vi "AB_Set_Library_Name_For_Destination.vi"(7 "allow empty string? (false)":bool, 8 "error in (no error)":errorcluster, 9 "library name":string, 10 "destination index":i32, 11 "destinations in":refnum<class "AB_Destination.lvclass">[](array[class])) -> (0 "error out":errorcluster, 2 "library name out":string, 3 "destinations out":refnum<class "AB_Destination.lvclass">[](array[class]))   [LabVIEW 2020]
uses:
  <vilib>/AppBuilder/AB_Classes/Destination/AB_Destination.lvclass
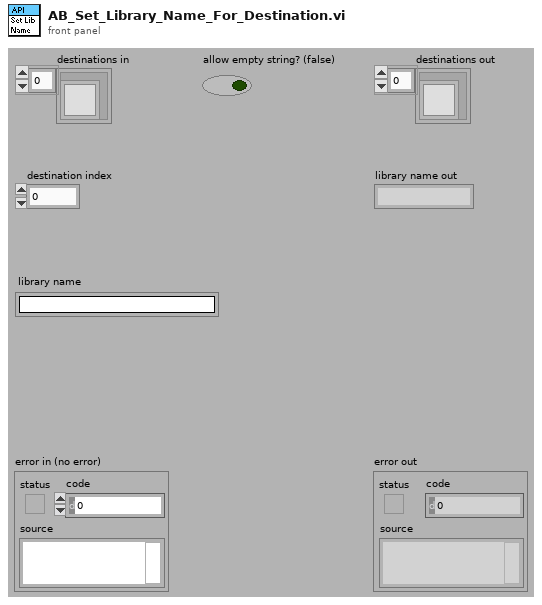
[diagram p1: front panel]
types:
  T1 = typedef "AB_Destination.ctl" = cluster{"destName":string, "path":path, "libraryName":string, "preserveHierarchy":bool, "eng_inBuild":bool, "eng_libraryReference":refnum<vi>, "eng_restictAddToNewLibrary":bool}
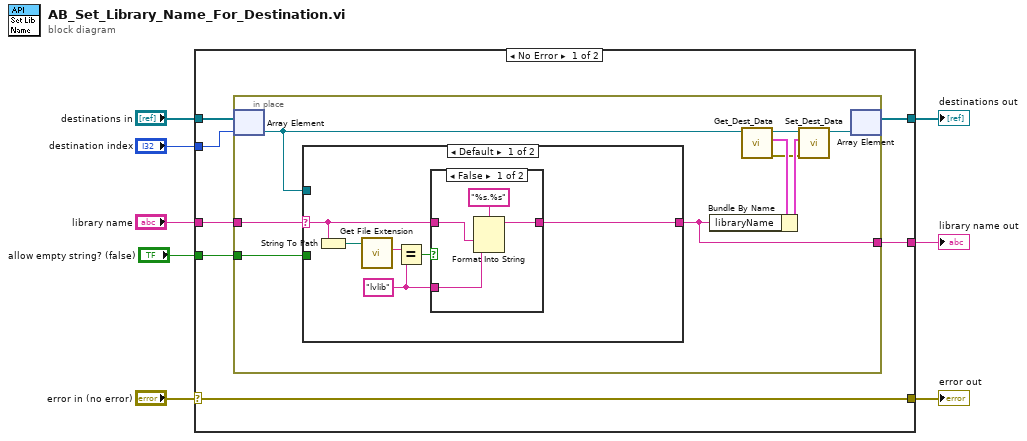
[diagram p0: block diagram]
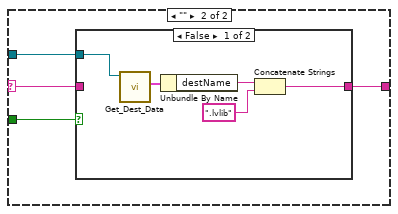
[diagram p3: hidden frame]
diagram:
  n1 = case shown="No Error" "error in (no error)" {
    selector: "error in (no error)" -> [w12 w47]
    tunnel: [w12 w47] -> w7
    tunnel: "destinations in" -> [w15 w46]
    tunnel: [w14 w46] -> w5
    tunnel: "destination index" -> [w13 _]
    tunnel: "library name" -> [w11 _]
    tunnel: "allow empty string? (false)" -> [w10 _]
    tunnel: [w9 _] -> w1
    frame No Error {
      n2 = in-place {
        in-place-border: w11 -> [w19]
        in-place-border: w10 -> [w17]
        in-place-border: [w16] -> w9
        n3 = in-place-array #1(w15, w13) -> (w18:refnum<class "AB_Destination.lvclass">)
        n4 = case shown="Default" w19 {
          selector: w19 -> [w26 w36]
          tunnel: [w25 w39] -> w16
          tunnel: w18 -> [_ w38]
          tunnel: w17 -> [_ w37]
          frame Default {
            w28 = "lvlib" ("y")
            n5 = String To Path(string=w26) -> (path=w29:path)
            n6 = call <vilib>:"Get File Extension.vi"("file"=w29) -> ("lowercase file extension"=w30:string)  [unwired: 1 in, 9 out]
            n7 = Equal?(x=w30, y=w28) -> (x = y?=w27:bool)
            n8 = case shown="False" w27 {
              tunnel: [w31 w35] -> w25
              tunnel: w26 -> [w33 w35]
              tunnel: w28 -> [w32 _]
              frame False {
                n9 = Format Into String(format string="%s.%s", w33, w32) -> (resulting string=w31:string)  [unwired: 2 in, 1 out]
              }
              frame True {
              }
            }
          }
          frame "" {
            n10 = case shown="False" w37 {
              tunnel: [w43 w45] -> w39
              tunnel: w38 -> [w40 _]
              tunnel: w36 -> [_ w45]
              frame False {
                n11 = call <vilib>:"Get_Dest_Data.vi"("Class in"=w40) -> ("destName"=w42:T1)  [unwired: 1 in, 9 out]
                n12 = Unbundle By Name(w42) -> ("destName"=w41:string)
                n13 = Concatenate Strings(w41, ".lvlib" ("y")) -> (w43:string)
              }
              frame True {
              }
            }
          }
        }
        n14 = call <vilib>:"Get_Dest_Data.vi"("Class in"=w18) -> ("error out"=w21:errorcluster, "destName"=w24:T1, "Class out"=w22:refnum<class "AB_Destination.lvclass">)  [unwired: 1 in, 7 out]
        n15 = Bundle By Name(cluster=w24, "libraryName"=w16) -> (w23:T1)
        n16 = call <vilib>:"Set_Dest_Data.vi"("error in (no error)"=w21, "destName"=w23, "Class in"=w22) -> ("Class out"=w20:refnum<class "AB_Destination.lvclass">)  [unwired: 8 out]
        n17 = in-place-array #1(w20) -> (w14:refnum<class "AB_Destination.lvclass">[])  [unwired: 1 out]
      }
    }
    frame Error {
    }
  }
  "error out" <- w7
  "destinations out" <- w5
  "library name out" <- w1
